vi "SecTomSec.vi"(11 "Sec":dbl) -> (3 "mSec":u32)   [LabVIEW 2013, in "Photometrics_CH-250_Cam.lvclass"]
uses:
  Photometrics_CH-250_Cam.lvclass
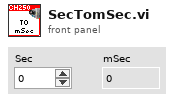
[diagram p1: front panel]
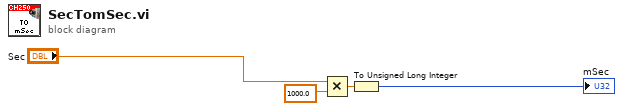
[diagram p0: block diagram]
diagram:
  n1 = Multiply(x="Sec", y=1000.0) -> (x*y=w1:dbl)
  n2 = To Unsigned Long Integer(number=w1) -> (unsigned 32bit integer=→"mSec":u32)
